vi "seria_if_some_read.vi"(0 "serial in":refnum<visa-resource-name>, 1 "error in (no error)":errorcluster) -> (2 "read buffer":string, 3 "serial out":refnum<visa-resource-name>, 4 "error out":errorcluster)   [LabVIEW 2016]
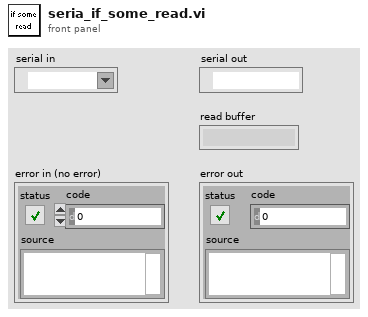
[diagram p1: front panel]
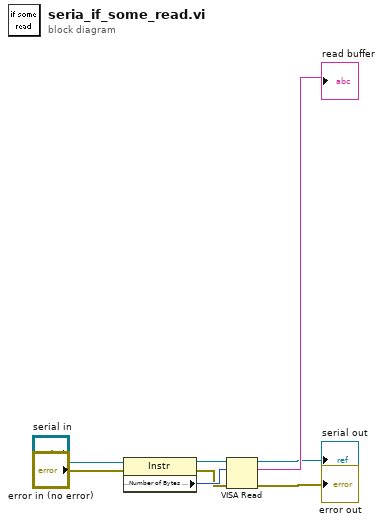
[diagram p0: block diagram]
diagram:
  n1 = property class="Instr"(reference="serial in", error in="error in (no error)") -> (reference out=w5:refnum<visa-resource-name>, error out=w6:errorcluster, "Serial Settings:Number of Bytes at Serial Port"=w7:u32)
  n2 = VISA Read(VISA resource name=w5, byte count=w7, error in (no error)=w6) -> (VISA resource name out=→"serial out":refnum<visa-resource-name>, read buffer=→"read buffer":string, error out=→"error out":errorcluster)  [unwired: 1 out]
